vi "get_signal_by_name.vi"(1 "Signal name":refnum<k21>, 2 "Signal list":refnum<k21>[](array[refnum]), 3 "Signal data":dbl[](array[numeric])) -> (0 "Signal":dbl)   [LabVIEW 2017]
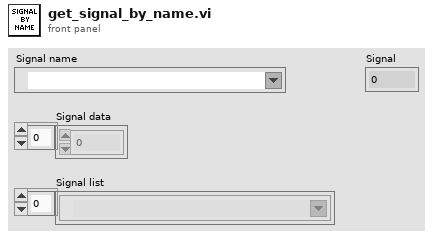
[diagram p1: front panel]
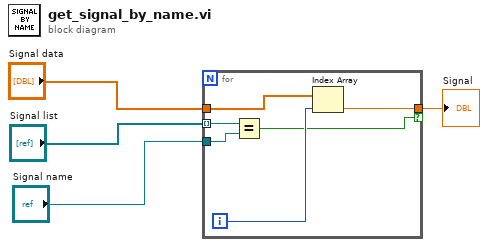
[diagram p0: block diagram]
diagram:
  n1 = for {
    tunnel: "Signal data" -> [w9]
    tunnel: "Signal list" -> [w10] mode=indexing
    tunnel: [w8] -> w4 if=w5
    tunnel: "Signal name" -> [w7]
    i -> [w6]
    n2 = Equal?(x=w10, y=w7) -> (x = y?=w5:bool)
    n3 = Index Array(array=w9, index=w6) -> (element=w8:dbl)
  }
  "Signal" <- w4
